vi "Destroy.vi"(0 "reference in":refnum<class "MyG#G3SubTempl.lvclass">, 5 "error in (no error)":errorcluster) -> (14 "reference out":refnum<class "MyG#G3SubTempl.lvclass">, 19 "error out":errorcluster)   [LabVIEW 2017, in "MyG#G3SubTempl.lvclass"]
doc: "Destructor."
uses:
  MyG#G3SubTempl.lvclass
  C:/Program Files/National Instruments/LabVIEW 2017/vi.lib/addons/_AddQ/G#Object/G#Object.lvclass
  MyG#G3Templ_class/MyG#G3Templ.lvclass
  <vilib>/addons/_AddQ/G#Object/G#Object.lvclass
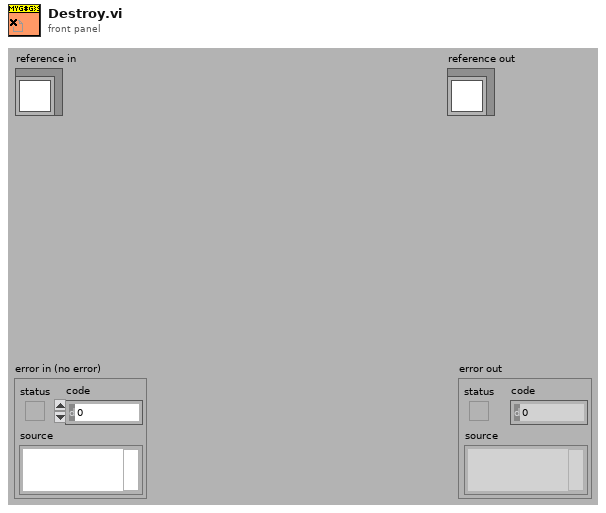
[diagram p1: front panel]
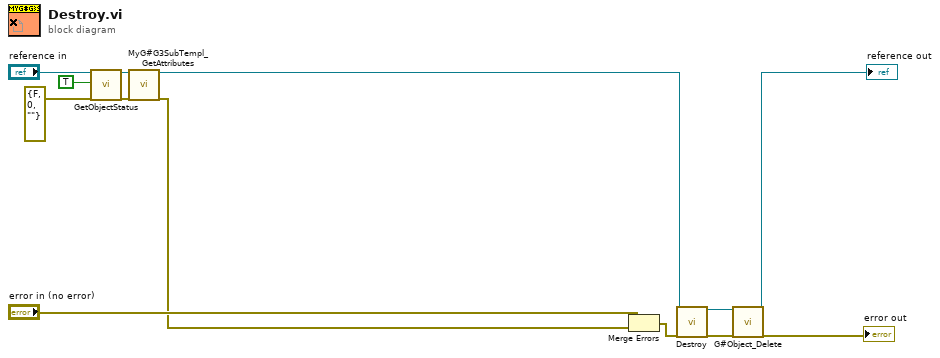
[diagram p0: block diagram]
diagram:
  n1 = call-dynamic "GetObjectStatus.vi"("reference in"="reference in", "simple info (F)"=TRUE ("simple info"), "error in (no error)"=errorcluster {"status"=FALSE, "code"=0, "source"=""}) -> ("reference out"=w4:refnum<class "MyG#G3SubTempl.lvclass">, "error out"=w5:errorcluster)  [unwired: 5 in, 10 out]
  n2 = call "MyG#G3SubTempl_GetAttributes.vi"("reference in"=w4, "error in (no error)"=w5) -> ("reference out"=w10:refnum<class "MyG#G3SubTempl.lvclass">, "error out"=w6:errorcluster)  [unwired: 14 in, 2 out]
  n3 = Merge Errors("error in (no error)", w6) -> (w11:errorcluster)
  n4 = call-parent "Destroy.vi"("reference in"=w10, "error in (no error)"=w11) -> ("reference out"=w8:refnum<class "MyG#G3SubTempl.lvclass">, "error out"=w9:errorcluster)  [unwired: 16 in]
  n5 = call <vilib>:"G#Object_Delete.vi"("reference in"=w8, "error in (no error)"=w9) -> ("reference out"=→"reference out":refnum<class "MyG#G3SubTempl.lvclass">, "error out"=→"error out":errorcluster)  [unwired: 16 in]
